vi "MSG.vi"() -> ()   [LabVIEW 2018]
panel:
  in  "MGS?":bool
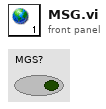
[diagram p1: front panel]
diagram:
